vi "Construct Actor Counts Message Cycles.vi"(8 "error in (no error)":errorcluster) -> (0 "error out":errorcluster, 2 "Final Count":refnum<notifier>, 3 "ActorCountsMessageCycles":refnum<class "ActorCountsMessageCycles.lvclass">)   [LabVIEW 2017, in "ActorCountsMessageCycles.lvclass"]
uses:
  ActorCountsMessageCycles.lvclass
  ActorCountsMessageCycles.lvclass/ActorCountsMessageCycles.ctl
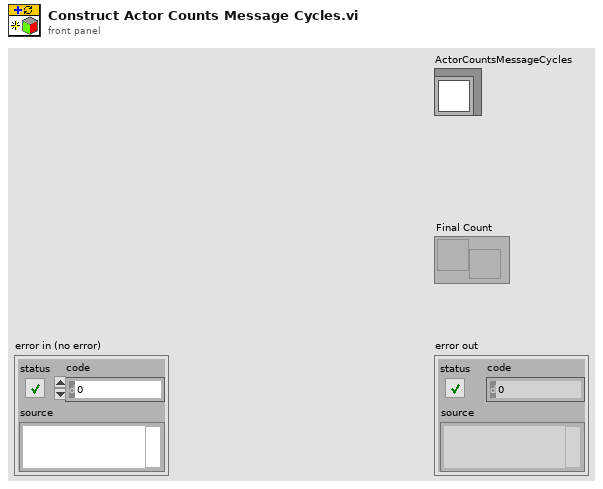
[diagram p1: front panel]
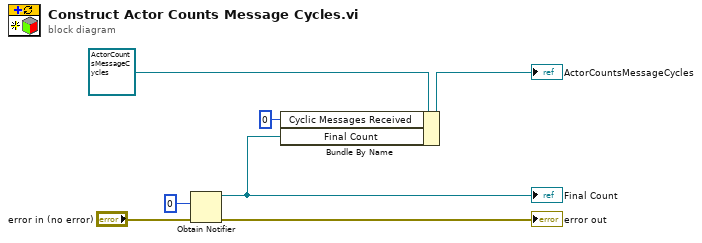
[diagram p0: block diagram]
diagram:
  n1 = Obtain Notifier(notification data type=u32 0, error in (no error)="error in (no error)") -> (notifier out=w4:refnum<notifier>, error out=→"error out":errorcluster)  [unwired: 2 in, 1 out]
  "Final Count" <- w4
  n2 = Bundle By Name(cluster=refnum<class "ActorCountsMessageCycles.lvclass"> refnum ("ActorCountsMessageCycles.lvclass"), "Cyclic Messages Received"=u32 0, "Final Count"=w4) -> (→"ActorCountsMessageCycles":refnum<class "ActorCountsMessageCycles.lvclass">)
